vi "U6 eDI Example.vi"() -> (0 "error out":errorcluster)   [LabVIEW 2020]
panel:
  in  "Address":string="1"
  in  "FirstFound":bool=TRUE
  out "State":bool
  in  "Channel":i32
  out "Error Message":string
  # "Reads 1 digital input using the UD easy function eDI."
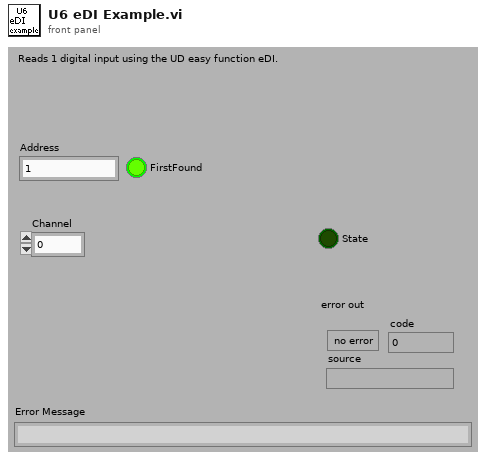
[diagram p1: front panel]
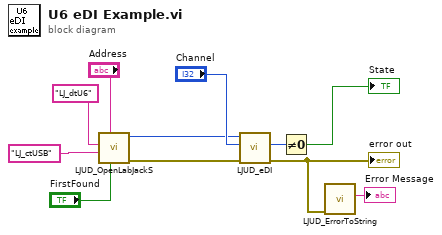
[diagram p0: block diagram]
diagram:
  n1 = call "LJUD_OpenLabJackS.vi"("FirstFound"="FirstFound", "Address"="Address", "ConnectionType"="LJ_ctUSB", "DeviceType"="LJ_dtU6") -> ("error out"=w2:errorcluster, "Handle"=w3:i32)  [unwired: 5 in, 1 out]
  n2 = call "LJUD_eDI.vi"("error in"=w2, "Channel"="Channel", "Handle In"=w3) -> ("error out"=w10:errorcluster, "State"=w8:i32)  [unwired: 6 in, 1 out]
  "error out" <- w10
  n3 = Not Equal To 0?(x=w8) -> (x != 0?=→"State":bool)
  n4 = call "LJUD_ErrorToString.vi"("error in"=w10) -> ("String"=→"Error Message":string)  [unwired: 10 in]
